vi "Write FlowControlValveCompensator.vi"(10 "FlowControlValveCompensator.lvclass":refnum<class "FlowControlValveCompensator.lvclass">, 11 "DualActingPneumaticCylinder in":refnum<class "DualActingPneumaticCylinder.lvclass">) -> (3 "DualActingPneumaticCylinder out":refnum<class "DualActingPneumaticCylinder.lvclass">)   [LabVIEW 2013, in "DualActingPneumaticCylinder.lvclass"]
uses:
  DualActingPneumaticCylinder.lvclass
  FlowControlValveCompensator/FlowControlValveCompensator.lvclass
  DualActingPneumaticCylinder.lvclass/DualActingPneumaticCylinder.ctl
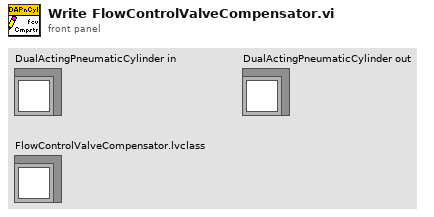
[diagram p1: front panel]
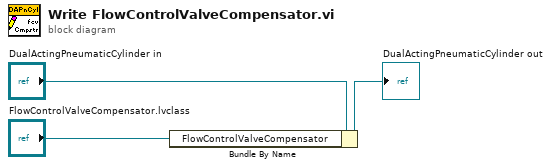
[diagram p0: block diagram]
diagram:
  n1 = Bundle By Name(cluster="DualActingPneumaticCylinder in", "FlowControlValveCompensator"="FlowControlValveCompensator.lvclass") -> (→"DualActingPneumaticCylinder out":refnum<class "DualActingPneumaticCylinder.lvclass">)
